vi "Command Parse.vi"(8 "error in (no error)":errorcluster, 9 "Read Buffer":string) -> (0 "error out":errorcluster)   [LabVIEW 2011]
uses:
  Enumerator/CmdType.ctl
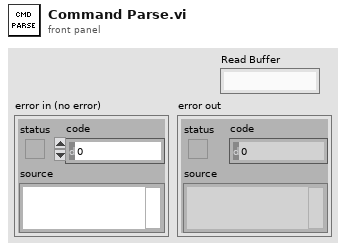
[diagram p1: front panel]
types:
  T1 = enum16{"Open", "R", "W", "R->W", "W->R", "Close"}
  T2 = typedef "CmdType.ctl" = enum16{"GetEventLog", "DelTransaction", "InvalidMessage", "RelayControl", "RelayOff", "RelayOn", "VaildMessage", "EventPolling", "StoppingWaiting", "PromptKeying-in"}
  T3 = enum16{"Obtain", "Enqueue", "Dequeue", "Release"}
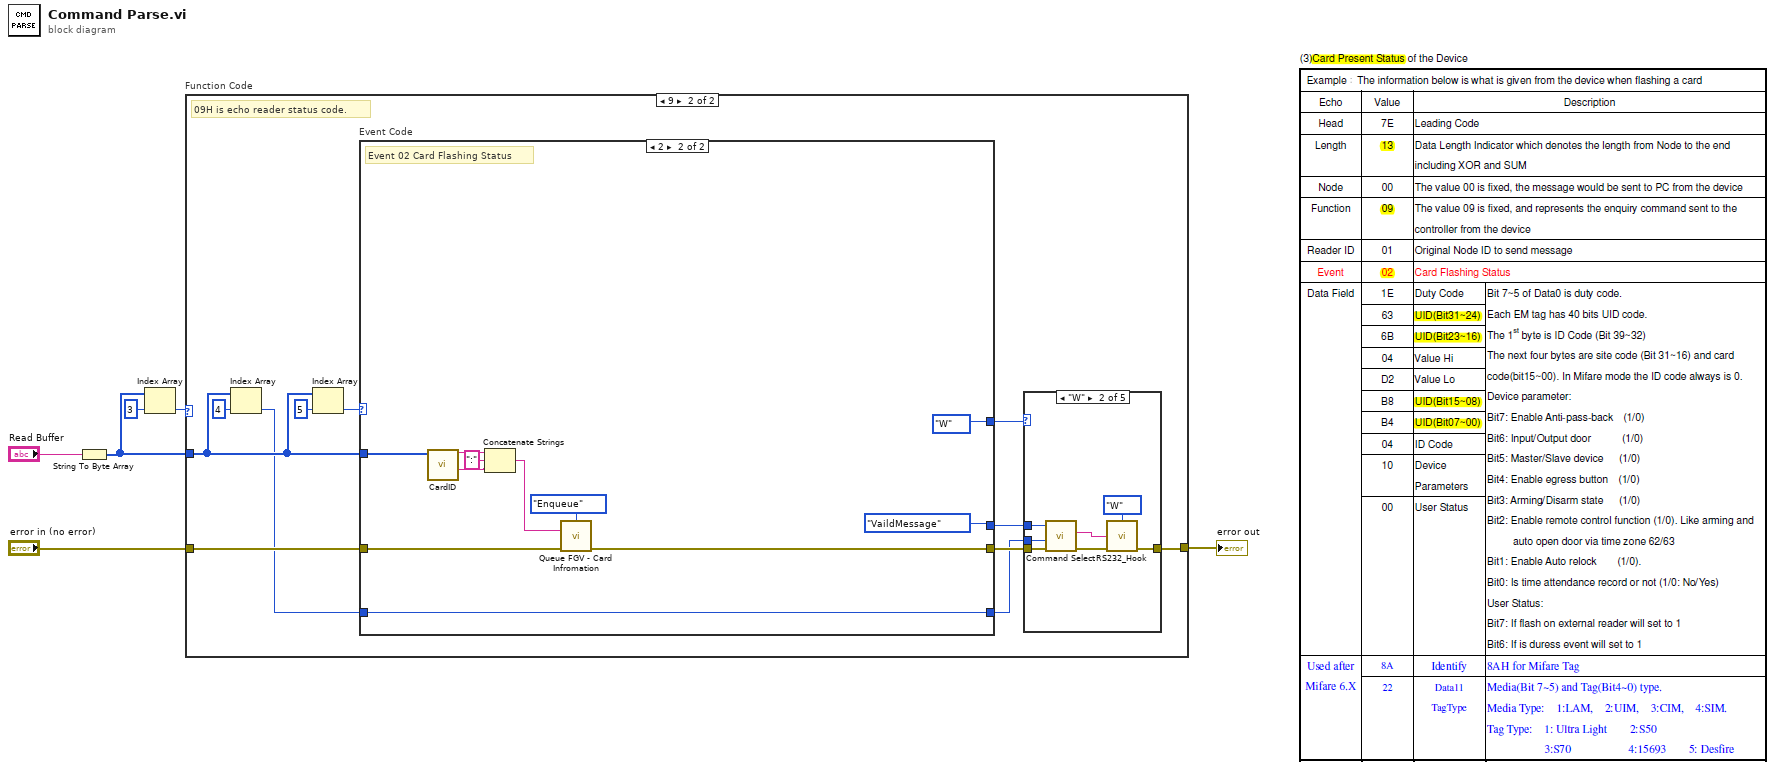
[diagram p0: block diagram]
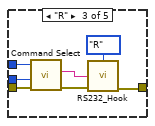
[diagram p4: hidden frame]
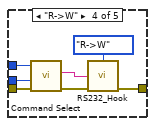
[diagram p5: hidden frame]
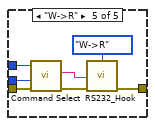
[diagram p6: hidden frame]
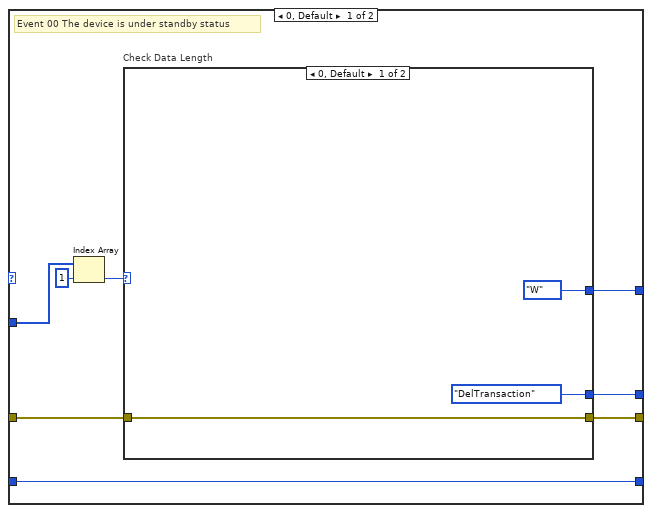
[diagram p7: hidden frame]
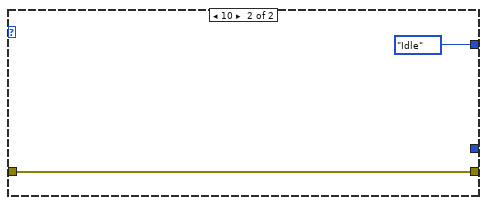
[diagram p8: hidden frame]
diagram:
  n1 = String To Byte Array(string="Read Buffer") -> (unsigned byte array=w1:u8[])
  n2 = Index Array(array=w1, index=3) -> (element=w3:u8)
  n3 = case "Function Code" shown="9" w3 {
    tunnel: "error in (no error)" -> [w7 w18]
    tunnel: [w7 w11] -> w6
    tunnel: w1 -> [_ w16]
    frame 4, Default {
      # "04H Command Acknowledge (ACK)"
    }
    frame 9 {
      # "09H is echo reader status code."
      n4 = Index Array(array=w16, index=4) -> (element=w13:u8)
      n5 = Index Array(array=w16, index=5) -> (element=w14:u8)
      n6 = case "Event Code" shown="2" w14 {
        tunnel: w18 -> [w55 w68]
        tunnel: w13 -> [w48 w69]
        tunnel: [w54 w67] -> w12
        tunnel: w16 -> [w51 w62]
        tunnel: [w48 w69] -> w10
        tunnel: [w50 CmdType."VaildMessage" ("CmdType")] -> w9
        tunnel: [w49 enum16{"Idle", "R", "W", "R->W", "W->R"}."W" ("Mode")] -> w8
        frame 0, Default {
          # "Event 00 The device is under standby status"
          n7 = Index Array(array=w51, index=1) -> (element=w52:u8)
          n8 = case "Check Data Length" shown="0, Default" w52 {
            tunnel: w55 -> [w58 w60]
            tunnel: [w58 w60] -> w54
            tunnel: [CmdType."DelTransaction" ("CmdType") _] -> w50
            tunnel: [enum16{"Idle", "R", "W", "R->W", "W->R"}."W" ("Mode") enum16{"Idle", "R", "W", "R->W", "W->R"}."Idle" ("Mode")] -> w49
            frame 0, Default {
            }
            frame 10 {
            }
          }
        }
        frame 2 {
          # "Event 02 Card Flashing Status"
          n9 = call "CardID.vi"("array in"=w62) -> ("Card ID"=w63:string, "Site ID"=w64:string)  [unwired: 9 in]
          n10 = Concatenate Strings(w64, ":" ("string"), w63) -> (w61:string)
          n11 = call "Queue FGV - Card Infromation.vi"("Mode"=T3."Enqueue", "Queue In"=w61, "error in (no error)"=w68) -> ("error out"=w67:errorcluster)  [unwired: 11 in, 1 out]
        }
      }
      n12 = case shown="\"W\"" w8 {
        tunnel: w12 -> [w19 w26 w33 w40 w47]
        tunnel: [w19 w21 w29 w35 w42] -> w11
        tunnel: w10 -> [_ w25 w32 w39 w46]
        tunnel: w9 -> [_ w24 w31 w38 w45]
        frame "Idle", Default {
        }
        frame "W" {
          n13 = call "Command Select.vi"("error in (no error)"=w26, "Node Id"=w25, "Cmd Type"=w24) -> ("error out"=w22:errorcluster, "Cmd Str"=w20:string)  [unwired: 7 in]
          n14 = call "RS232_Hook.vi"("Mode"=T1."W", "data in"=w20, "error in"=w22) -> ("error out"=w21:errorcluster)  [unwired: 11 in, 1 out]
        }
        frame "R" {
          n15 = call "Command Select.vi"("error in (no error)"=w33, "Node Id"=w32, "Cmd Type"=w31) -> ("error out"=w30:errorcluster, "Cmd Str"=w27:string)  [unwired: 7 in]
          n16 = call "RS232_Hook.vi"("Mode"=T1."R", "data in"=w27, "error in"=w30) -> ("error out"=w29:errorcluster)  [unwired: 11 in, 1 out]
        }
        frame "R->W" {
          n17 = call "Command Select.vi"("error in (no error)"=w40, "Node Id"=w39, "Cmd Type"=w38) -> ("error out"=w36:errorcluster, "Cmd Str"=w34:string)  [unwired: 7 in]
          n18 = call "RS232_Hook.vi"("Mode"=T1."R->W", "data in"=w34, "error in"=w36) -> ("error out"=w35:errorcluster)  [unwired: 11 in, 1 out]
        }
        frame "W->R" {
          n19 = call "Command Select.vi"("error in (no error)"=w47, "Node Id"=w46, "Cmd Type"=w45) -> ("error out"=w43:errorcluster, "Cmd Str"=w41:string)  [unwired: 7 in]
          n20 = call "RS232_Hook.vi"("Mode"=T1."W->R", "data in"=w41, "error in"=w43) -> ("error out"=w42:errorcluster)  [unwired: 11 in, 1 out]
        }
      }
    }
  }
  "error out" <- w6
